vi "Add Sequence.vi"(8 "error in (no error)":errorcluster, 10 "Transition Sequence":T1[](array[typedef]), 11 "Queue in":refnum<queue>) -> (0 "error out":errorcluster, 3 "Queue out":refnum<queue>)   [LabVIEW 2017, in "Shared Variables CD 2.0 Configuration.lvlib"]
doc: "Add a sequence of states to execute"
uses:
  Shared Variables CD 2.0 Configuration.lvlib
  Channel Configuration States.ctl
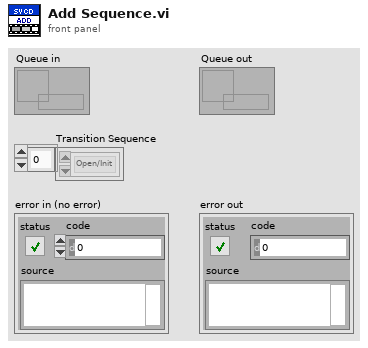
[diagram p1: front panel]
types:
  T1 = typedef "Shared Variables CD 2.0 Configuration.lvlib/Channel Configuration States.ctl" = enum16{"Open/Init", "Start Update", "Get VS Channels", "Get Available Ch from Target", "Wait On User Action", "Update Target Tree", "Update VS Trees", "Update Done", "Create VS Channels", "Remove VS Channels", "Error", "Close"}
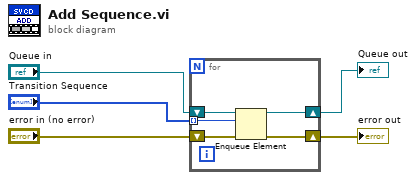
[diagram p0: block diagram]
diagram:
  n1 = for {
    shift-right: [w9] -> w2
    shift-left: "error in (no error)" -> [w10]
    shift-right: [w7] -> w4
    shift-left: "Queue in" -> [w8]
    tunnel: "Transition Sequence" -> [w6] mode=indexing
    n2 = Enqueue Element(queue=w8, element=w6, error in (no error)=w10) -> (queue out=w7:refnum<queue>, error out=w9:errorcluster)  [unwired: 1 in, 1 out]
  }
  "Queue out" <- w4
  "error out" <- w2
